vi "Get Server Address.vi"(11 "OOP Server in":refnum<class "TempController_server.lvclass">) -> (2 "Server Address":string, 3 "OOP Server out":refnum<class "TempController_server.lvclass">)   [LabVIEW 2019, in "TempController_server.lvlib" / "TempController_server.lvclass"]
uses:
  TempController_server.lvclass
  TempController_server.lvclass/TempController_server.ctl
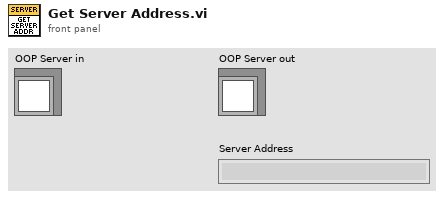
[diagram p1: front panel]
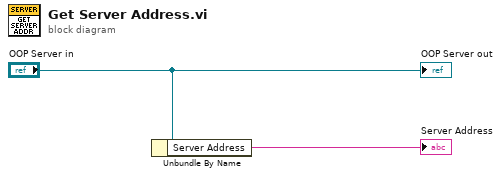
[diagram p0: block diagram]
diagram:
  n1 = Unbundle By Name("OOP Server in") -> ("Server Address"=→"Server Address":string)
  "OOP Server out" <- "OOP Server in"
